vi "Mappa AI DI PLC_1.vi"(0 "USCITE PLC":T1, 1 "MBit read":bool[](array[boolean]), 2 "MW read":dbl[](array[numeric]), 3 "M real read":dbl[](array[numeric]), 4 "Array DB bit":bool[](array[boolean]), 5 "DB WORD":dbl[](array[numeric]), 7 "DB REAL":dbl[](array[numeric])) -> (14 "STATO PLC":T4)   [LabVIEW 2019]
uses:
  STATO PLC 1.ctl
  Uscite PLC 1.ctl
  controls/statoAO_plc_1.ctl
  StatoDO_PLC_1.ctl
panel:
  # "StatoDO_PLC.ctlUSCITE PLC : TYPE DEF"
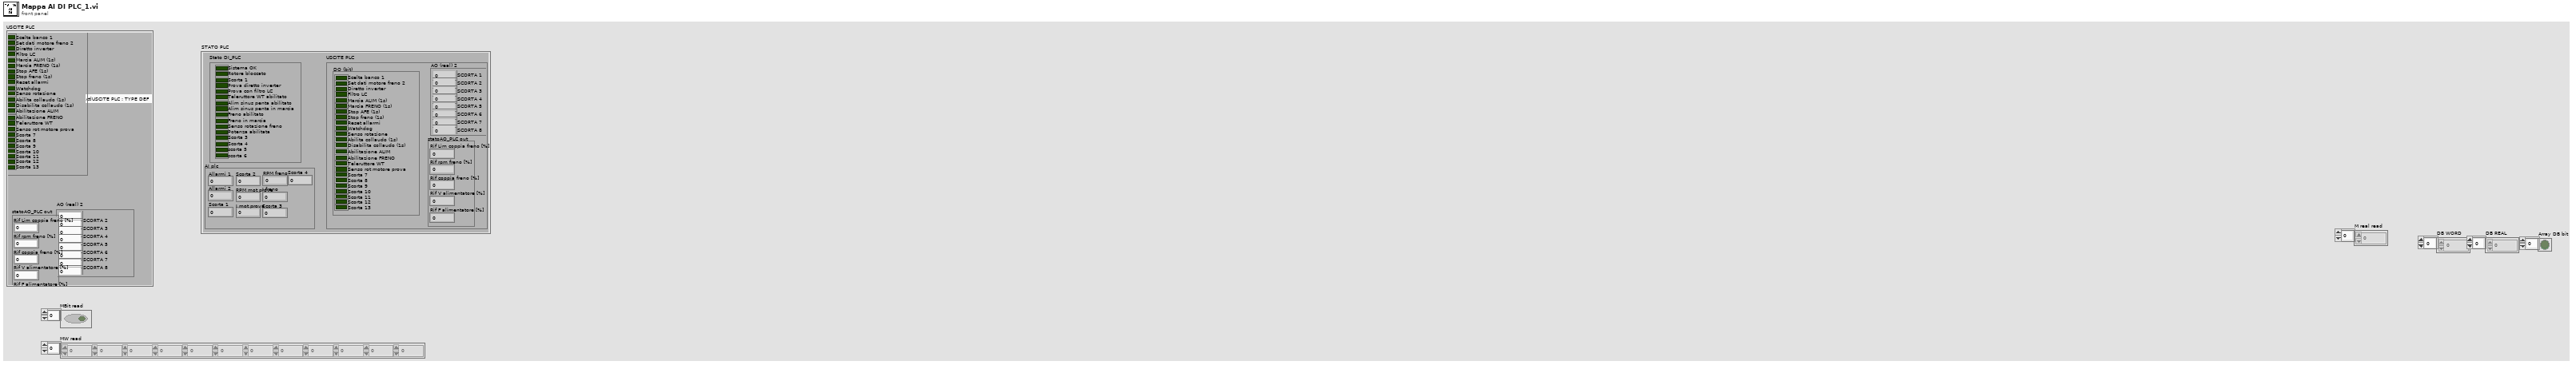
[diagram p1: front panel]
types:
  T1 = typedef "Uscite PLC 1.ctl" = cluster{"AO (real) 2":cluster{"SCORTA 1":dbl, "SCORTA 2":dbl, "SCORTA 3":dbl, "SCORTA 4":dbl, "SCORTA 5":dbl, "SCORTA 6":dbl, "SCORTA 7":dbl, "SCORTA 8":dbl}, "statoAO_PLC out":T2, "DO (bit)":T3}
  T2 = typedef "statoAO_plc_1.ctl" = cluster{"Rif Lim coppia freno [%]":dbl, "Rif rpm freno [%]":dbl, "Rif coppia freno [%]":dbl, "Rif V alimentatore [%]":dbl, "Rif F alimentatore [%]":dbl}
  T3 = typedef "StatoDO_PLC_1.ctl" = cluster{"Scelta banco 1":bool, "Set dati motore freno 2":bool, "Diretto inverter":bool, "Filtro LC":bool, "Marcia ALIM (1s)":bool, "Marcia FRENO (1s)":bool, "Stop AFE (1s)":bool, "Stop freno (1s)":bool, "Reset allarmi":bool, "Watchdog":bool, "Senso rotazione":bool, "Abilita collaudo (1s)":bool, "Disabilita collaudo (1s)":bool, "Abilitazione ALIM":bool, "Abilitazione FRENO":bool, "Teleruttore WT":bool, "Senso rot motore prova":bool, "Scorta 7":bool, "Scorta 8":bool, "Scorta 9":bool, "Scorta 10":bool, "Scorta 11":bool, "Scorta 12":bool, "Scorta 13":bool}
  T4 = typedef "STATO PLC 1.ctl" = cluster{"USCITE PLC":T1, "Stato DI_PLC":cluster{"Sistema OK":bool, "Rotore bloccato":bool, "Scorta 1":bool, "Prova diretto inverter":bool, "Prova con filtro LC":bool, "Teleruttore WT abilitato":bool, "Alim sinus penta abilitato":bool, "Alim sinus penta in marcia":bool, "Freno abilitato":bool, "Freno in marcia":bool, "Senso rotazione freno":bool, "Potenza abilitata":bool, "Scorta 3":bool, "Scorta 4":bool, "scorta 5":bool, "scorta 6":bool}, "AI plc":cluster{"Allarmi 1":dbl, "Allarmi 2":dbl, "Scorta 1":dbl, "Scorta 2":dbl, "RPM mot prova":dbl, "I mot prova":dbl, "RPM freno":dbl, "I freno":dbl, "Scorta 3":dbl, "Scorta 4":dbl}}
  T5 = cluster{"MBit read[0]":bool, "MBit read[1]":bool, "MBit read[2]":bool, "MBit read[3]":bool, "MBit read[4]":bool, "MBit read[5]":bool, "MBit read[6]":bool, "MBit read[7]":bool, "MBit read[8]":bool, "MBit read[9]":bool, "MBit read[10]":bool, "MBit read[11]":bool, "MBit read[12]":bool, "MBit read[13]":bool, "MBit read[14]":bool, "MBit read[15]":bool}
  T6 = cluster{"MW read[0]":dbl, "MW read[1]":dbl, "MW read[2]":dbl, "MW read[3]":dbl, "MW read[4]":dbl, "MW read[5]":dbl, "MW read[6]":dbl, "MW read[7]":dbl, "MW read[8]":dbl, "MW read[9]":dbl}
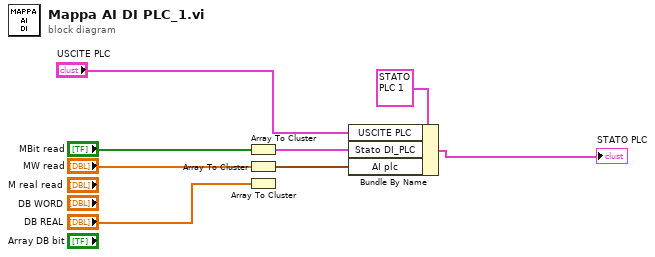
[diagram p0: block diagram]
diagram:
  n1 = Array To Cluster(array="MBit read") -> (cluster=w5:T5)
  n2 = Array To Cluster(array="MW read") -> (cluster=w2:T6)
  n3 = Array To Cluster(array="DB REAL") -> ()  [unwired: 1 out]
  n4 = Bundle By Name(cluster=T4 {"USCITE PLC"={"AO (real) 2"={"SCORTA 1"=0.0, "SCORTA 2"=0.0, "SCORTA 3"=0.0, "SCORTA 4"=0.0, "SCORTA 5"=0.0, "SCORTA 6"=0.0, "SCORTA 7"=0.0, "SCORTA 8"=0.0}, "statoAO_PLC out"={"Rif Lim coppia freno [%]"=0.0, "Rif rpm freno [%]"=0.0, "Rif coppia freno [%]"=0.0, "Rif V alimentatore [%]"=0.0, "Rif F alimentatore [%]"=0.0}, "DO (bit)"={"Scelta banco 1"=FALSE, "Set dati motore freno 2"=FALSE, "Diretto inverter"=FALSE, "Filtro LC"=FALSE, "Marcia ALIM (1s)"=FALSE, "Marcia FRENO (1s)"=FALSE, "Stop AFE (1s)"=FALSE, "Stop freno (1s)"=FALSE, "Reset allarmi"=FALSE, "Watchdog"=FALSE, "Senso rotazione"=FALSE, "Abilita collaudo (1s)"=FALSE, "Disabilita collaudo (1s)"=FALSE, "Abilitazione ALIM"=FALSE, "Abilitazione FRENO"=FALSE, "Teleruttore WT"=FALSE, "Senso rot motore prova"=FALSE, "Scorta 7"=FALSE, "Scorta 8"=FALSE, "Scorta 9"=FALSE, "Scorta 10"=FALSE, "Scorta 11"=FALSE, "Scorta 12"=FALSE, "Scorta 13"=FALSE}}, "Stato DI_PLC"={"Sistema OK"=FALSE, "Rotore bloccato"=FALSE, "Scorta 1"=FALSE, "Prova diretto inverter"=FALSE, "Prova con filtro LC"=FALSE, "Teleruttore WT abilitato"=FALSE, "Alim sinus penta abilitato"=FALSE, "Alim sinus penta in marcia"=FALSE, "Freno abilitato"=FALSE, "Freno in marcia"=FALSE, "Senso rotazione freno"=FALSE, "Potenza abilitata"=FALSE, "Scorta 3"=FALSE, "Scorta 4"=FALSE, "scorta 5"=FALSE, "scorta 6"=FALSE}, "AI plc"={"Allarmi 1"=0.0, "Allarmi 2"=0.0, "Scorta 1"=0.0, "Scorta 2"=0.0, "RPM mot prova"=0.0, "I mot prova"=0.0, "RPM freno"=0.0, "I freno"=0.0, "Scorta 3"=0.0, "Scorta 4"=0.0}} ("STATO PLC"), "USCITE PLC"="USCITE PLC", "Stato DI_PLC"=w5, "AI plc"=w2) -> (→"STATO PLC":T4)
